vi "WriteObjects.vi"(8 "Error In":errorcluster, 10 "Objects":T1(array[cluster]), 11 "object in":refnum<class "TAFConfiguration.lvclass">) -> (0 "Error Out":errorcluster, 3 "object out":refnum<class "TAFConfiguration.lvclass">)   [LabVIEW 2021, in "TAF Proj Document Type.lvlib" / "TAFConfiguration.lvclass"]
uses:
  <vilib>/Wovalab/AntiDoc/Document Type/Add-ons/LabVIEW TAF Project/TAFConfiguration/TAFConfiguration.lvclass
  <vilib>/Wovalab/AntiDoc/Document Type/Add-ons/LabVIEW TAF Project/TAFConfiguration/TAFConfiguration.lvclass/TAFConfiguration.ctl
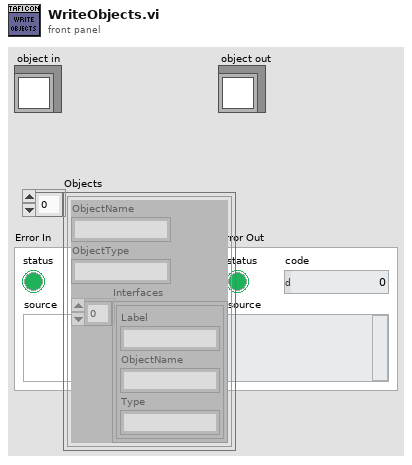
[diagram p1: front panel]
types:
  T1 = cluster{"ObjectName":string, "ObjectType":string, "Interfaces":cluster{"Label":string, "ObjectName":string, "Type":string}[]}[]
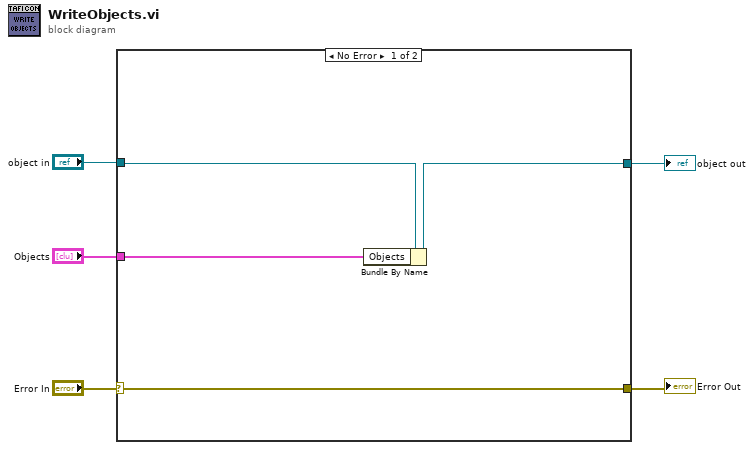
[diagram p0: block diagram]
diagram:
  n1 = case shown="No Error" "Error In" {
    selector: "Error In" -> [w8 w11]
    tunnel: [w8 w11] -> w4
    tunnel: [w6 w10] -> w2
    tunnel: "object in" -> [w7 w10]
    tunnel: "Objects" -> [w9 _]
    frame No Error {
      n2 = Bundle By Name(cluster=w7, "Objects"=w9) -> (w6:refnum<class "TAFConfiguration.lvclass">)
    }
    frame Error {
    }
  }
  "Error Out" <- w4
  "object out" <- w2
